vi "position from parameters and phase.vi"() -> ()   [LabVIEW 2017]
panel:
  out "size(s) 2":i32[](array[numeric])
  out "size(s)":i32
  out "derivatives (i,j) =":dbl[][](array[numeric])
  in  "phase":dbl
  in  "theta_axis":dbl
  in  "b":dbl
  in  "a":dbl
  in  "L":dbl
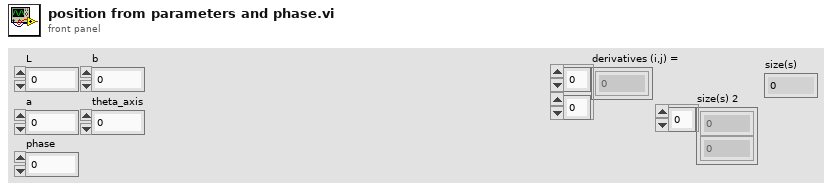
[diagram p1: front panel]
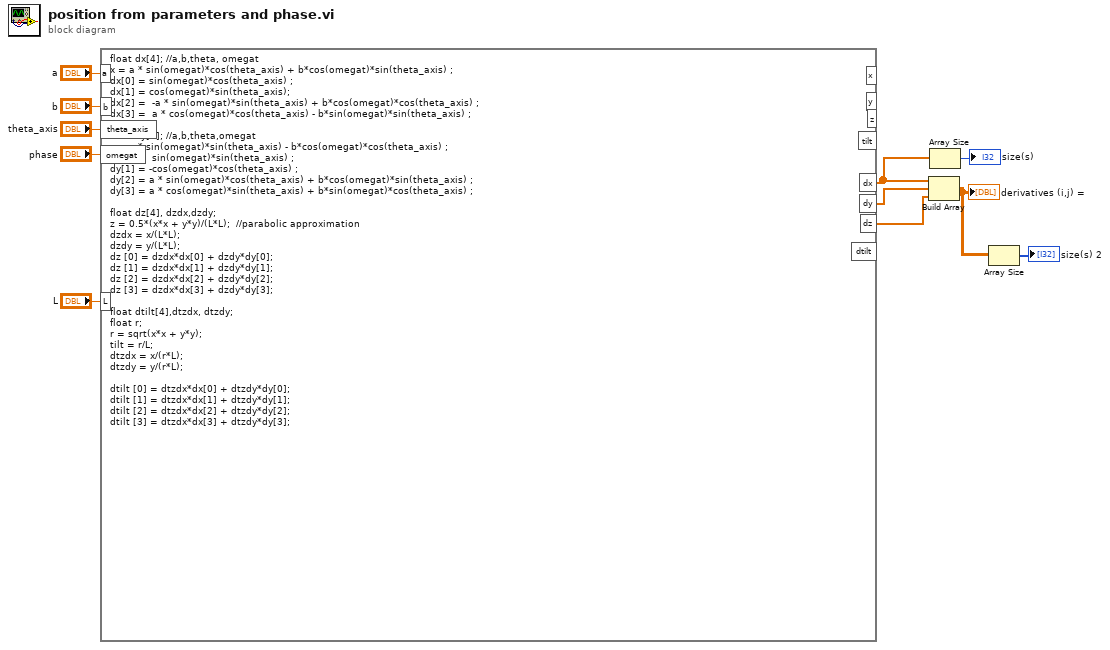
[diagram p0: block diagram]
diagram:
  n1 = formula code="float dx[4]; //a,b,theta, omegat\nx = a * sin(omegat)*cos(theta_axis) + b*cos(omegat)*sin(theta_axis) ;\ndx[0] = sin(omegat)*cos(theta_axis) ;\ndx[1] = cos(omegat)*sin(theta_axis);\ndx[2] =  -a * sin(omegat)*sin(theta_axis) + b*cos(omegat)*cos(theta_axis) ;\ndx[3] =  a * cos(omegat)*cos(theta_axis) - b*sin(omegat)*sin(theta_axis) ;\n\nfloat dy[4]; //a,b,theta,omegat\ny = a * sin(omegat)*sin(theta_axis) - b*cos(omegat)*cos(theta_axis) ;\ndy[0] =  sin(omegat)*sin(theta_axis) ;\ndy[1] = -cos(omegat)*cos(theta_axis) ;\ndy[2] = a * sin(omegat)*cos(theta_axis) + b*cos(omegat)*sin(theta_axis) ;\ndy[3] = a * cos(omegat)*sin(theta_axis) + b*sin(omegat)*cos(theta_axis) ;\n\nfloat dz[4], dzdx,dzdy;\nz = 0.5*(x*x + y*y)/(L*L);  //parabolic approximation\ndzdx = x/(L*L);\ndzdy = y/(L*L);\ndz [0] = dzdx*dx[0] + dzdy*dy[0];\ndz [1] = dzdx*dx[1] + dzdy*dy[1];\ndz [2] = dzdx*dx[2] + dzdy*dy[2];\ndz [3] = dzdx*dx[3] + dzdy*dy[3];\n\nfloat dtilt[4],dtzdx, dtzdy;\nfloat r;\nr = sqrt(x*x + y*y);\ntilt = r/L;\ndtzdx = x/(r*L);\ndtzdy = y/(r*L);\n\ndtilt [0] = dtzdx*dx[0] + dtzdy*dy[0];\ndtilt [1] = dtzdx*dx[1] + dtzdy*dy[1];\ndtilt [2] = dtzdx*dx[2] + dtzdy*dy[2];\ndtilt [3] = dtzdx*dx[3] + dtzdy*dy[3];"("omegat"="phase", "a"="a", "b"="b", "L"="L", "theta_axis"="theta_axis") -> ("dx"=w4:dbl[], "dy"=w5:dbl[], "dz"=w6:dbl[])  [unwired: 5 out]
  n2 = Build Array(w4, w5, w6) -> (w3:dbl[][])
  "derivatives (i,j) =" <- w3
  n3 = Array Size(array=w4) -> (size(s)=→"size(s)":i32)
  n4 = Array Size(array=w3) -> (size(s)=→"size(s) 2":i32[])
